vi "Flow and Pressure Sensors V5.vi"() -> ()   [LabVIEW 2018]
uses:
  <vilib>/Instr/_visa.llb/VISA Configure Serial Port (Instr).vi
panel:
  out "Flow Sensor Waveform":dynamicdata(graph)
  out "Pressure Sensor Waveform":dynamicdata(graph)
  out "Data Write Error Out":errorcluster
  out "Raw Data":string
  out "Pressure Output":string
  in  "File Name":string="default"
  in  "File Location":path
  out "Serial Settings:Number of Bytes at Serial Port":u32
  out "Close Error":errorcluster
  out "Data Format Error":errorcluster
  out "Flow Output":string
  in  "?":bool
  in  "COM":refnum<visa-resource-name>
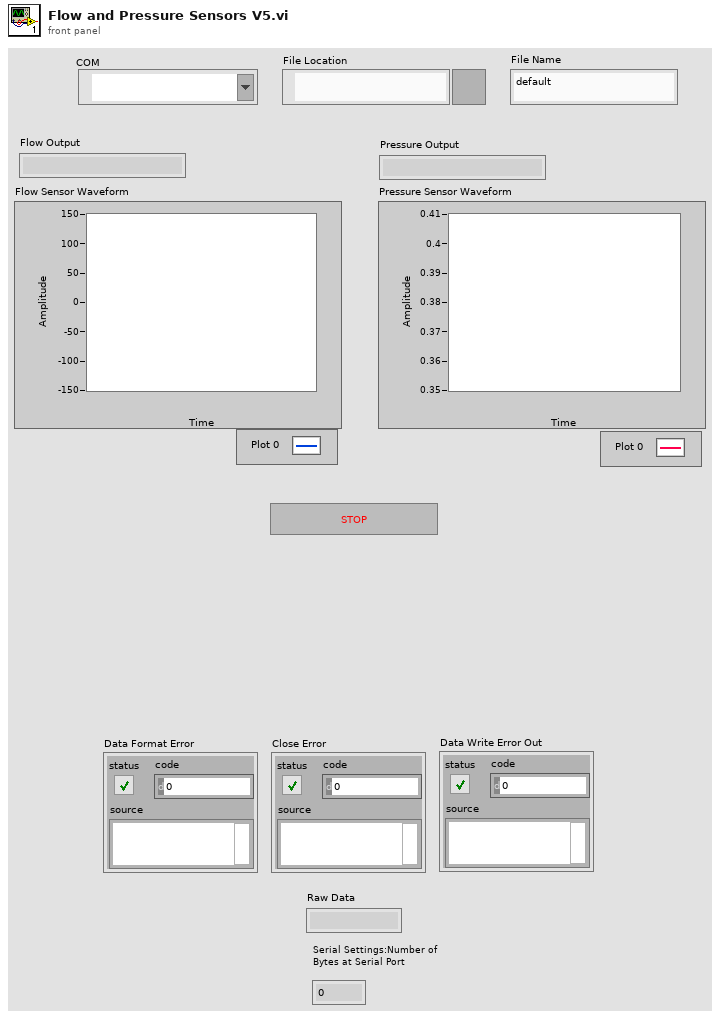
[diagram p1: front panel]
types:
  T1 = enum16{"open", "replace", "create", "open or create", "replace or create", "replace or create with confirmation"}
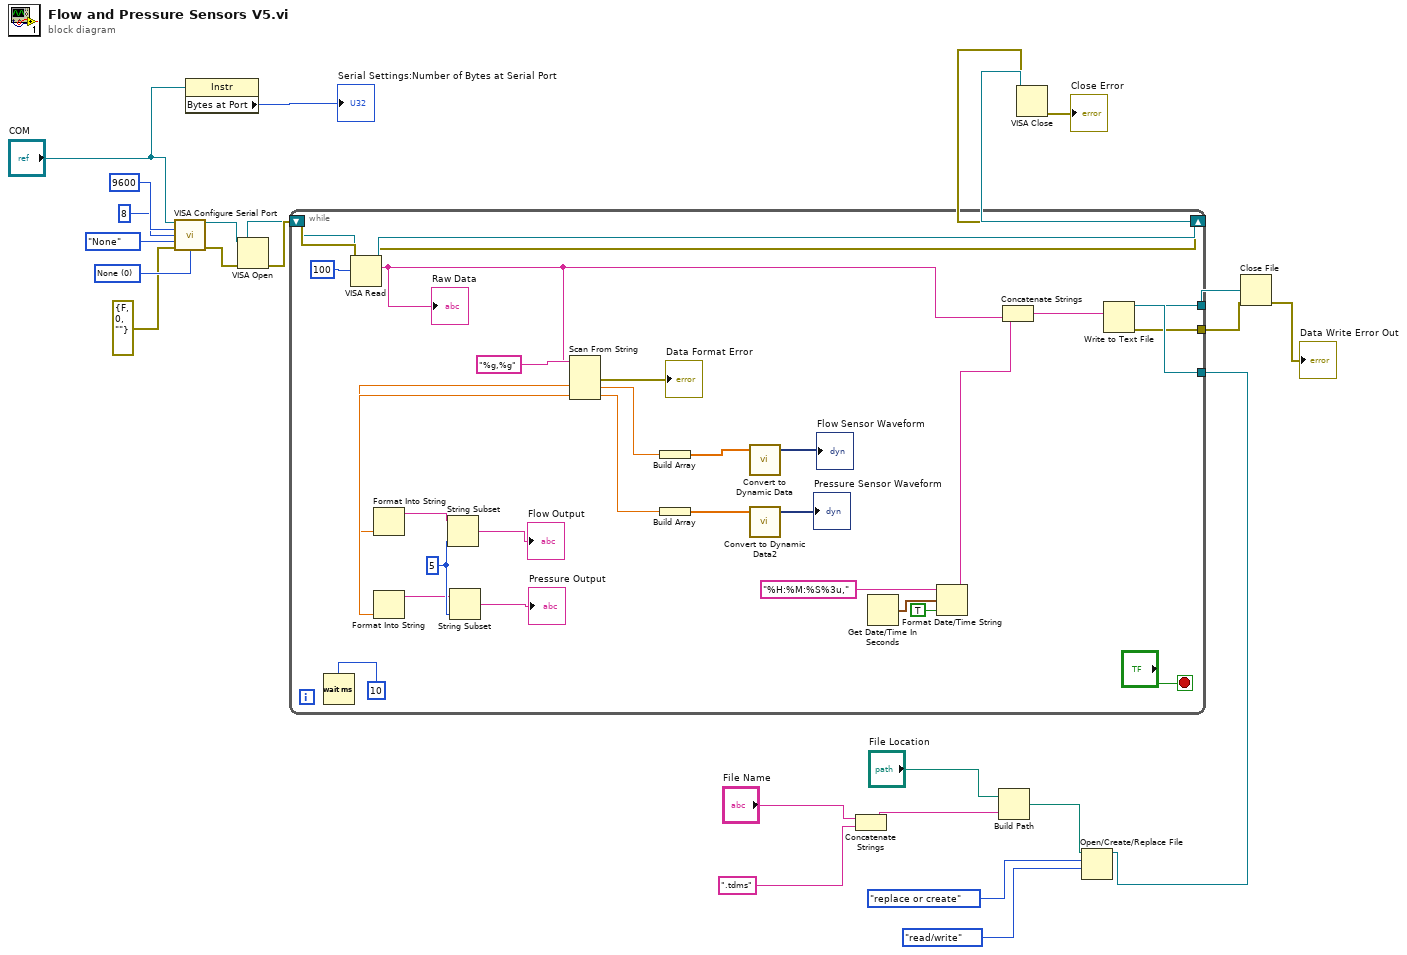
[diagram p0: block diagram]
diagram:
  w21 = u16 0 items=["None", "XON/XOFF", "RTS/CTS", "XON/XOFF & RTS/CTS", "DTR/DSR", "XON/XOFF & DTR/DSR"] ("flow control (0:none)")
  n1 = call-poly "VISA Configure Serial Port"("VISA resource name"="COM", "baud rate (9600)"=u32 9600, "data bits (8)"=u16 8, "parity (0:none)"=enum16{"None", "Odd", "Even", "Mark", "Space"}."None", "error in (no error)"=errorcluster {"status"=FALSE, "code"=0, "source"=""}, "flow control (0:none)"=w21) -> ("VISA resource name out"=w17:refnum<visa-resource-name>, "error out"=w20:errorcluster)  [unwired: 8 in]
  n2 = property class="Instr"(reference="COM") -> ("Bytes at Port"=→"Serial Settings:Number of Bytes at Serial Port":u32)  [unwired: 1 in, 2 out]
  n3 = VISA Open(error in (no error)=w20, VISA resource name=w17) -> (error out=w19:errorcluster)  [unwired: 3 in, 1 out]
  n4 = Concatenate Strings("File Name", ".tdms" ("time format string (%c)")) -> (w4:string)
  n5 = Build Path(base path="File Location", name or relative path=w4) -> (appended path=w10:path)
  n6 = Open/Create/Replace File(file path (use dialog)=w10, operation (0:open)=T1."replace or create", access (0:read/write)=enum16{"read/write", "read-only", "write-only"}."read/write") -> (refnum out=w7:refnum<file>)  [unwired: 3 in, 2 out]
  n7 = while {
    shift-right: [w49] -> w15
    shift-left: w19 -> [w53]
    shift-right: [w50] -> w16
    shift-left: w17 -> [w51]
    tunnel: w7 -> [w32]
    tunnel: [w28] -> w3
    tunnel: [w27] -> w1
    stop <- "?" stop-if-true
    w38 = u32 5 ("byte count")
    n8 = Wait (ms)(milliseconds to wait=u32 10) -> ()  [unwired: 1 out]
    n9 = VISA Read(VISA resource name=w51, byte count=u32 100, error in (no error)=w53) -> (VISA resource name out=w50:refnum<visa-resource-name>, read buffer=w30:string, error out=w49:errorcluster)  [unwired: 1 out]
    "Raw Data" <- w30
    n10 = Scan From String(format string="%g,%g", input string=w30) -> (error out=→"Data Format Error":errorcluster, output 1=w33:dbl, output 2=w40:dbl)  [unwired: 4 in, 2 out]
    n11 = Format Into String(w33) -> (resulting string=w39:string)  [unwired: 3 in, 1 out]
    n12 = Format Into String(w40) -> (resulting string=w37:string)  [unwired: 3 in, 1 out]
    n13 = String Subset(string=w39, length (rest)=w38) -> (substring=→"Flow Output":string)  [unwired: 1 in]
    n14 = String Subset(string=w37, length (rest)=w38) -> (substring=→"Pressure Output":string)  [unwired: 1 in]
    n15 = Build Array(w33) -> (w34:dbl[])
    n16 = Build Array(w40) -> (w44:dbl[])
    n17 = call "Convert to Dynamic Data"("Array"=w34) -> ("Dynamic Data Type"=→"Flow Sensor Waveform":dynamicdata)  [unwired: 3 in]
    n18 = call "Convert to Dynamic Data2"("Array"=w44) -> ("Dynamic Data Type"=→"Pressure Sensor Waveform":dynamicdata)  [unwired: 3 in]
    n19 = Get Date/Time In Seconds() -> (seconds since 1Jan1904=w43:timestamp)
    n20 = Format Date/Time String(time format string (%c)="%H:%M:%S%3u,", seconds (now)=w43, UTC format=TRUE) -> (date/time string=w31:string)
    n21 = Concatenate Strings(w31, w30) -> (w29:string)
    n22 = Write to Text File(file (use dialog)=w32, text=w29) -> (refnum out=w28:refnum<file>, error out=w27:errorcluster)  [unwired: 2 in, 1 out]
  }
  n23 = VISA Close(VISA resource name=w16, error in (no error)=w15) -> (error out=→"Close Error":errorcluster)
  n24 = Close File(refnum=w3, error in=w1) -> (error out=→"Data Write Error Out":errorcluster)  [unwired: 1 out]
